vi "Get RPC getCANDatafromrgrpcServer_clientRequester_getIDFormServer __Input.vi"(8 "error in (no error)":errorcluster, 11 "gRPCid in":T1) -> (0 "error out":errorcluster, 2 "Message Data":T2, 3 "gRPCid out":T1)   [LabVIEW 2020, in "server12.lvlib" / "server12.lvclass"]
uses:
  server12.lvclass
  gRPC lvSupport/Server API/typeDefs/grpcId.ctl
  server12.lvclass/server12.ctl
  gRPC lvSupport/gprc-lvsupport.lvlib
  RPC Messages/getCANDatafromrgrpcServer_inputSettings/getCANDatafromrgrpcServer_inputSettings_Data.ctl
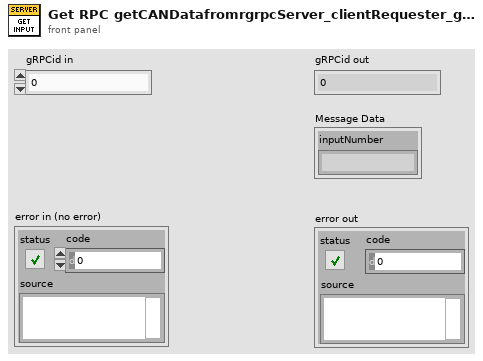
[diagram p1: front panel]
types:
  T1 = typedef "server12.lvlib/gprc-lvsupport.lvlib/grpcId.ctl" = u64
  T2 = typedef "server12.lvlib/server12.lvclass/getCANDatafromrgrpcServer_inputSettings_Data.ctl" = cluster{"inputNumber":string}
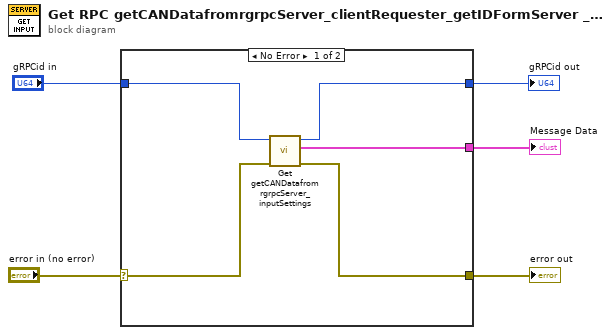
[diagram p0: block diagram]
diagram:
  n1 = case shown="No Error" "error in (no error)" {
    selector: "error in (no error)" -> [w10 w11]
    tunnel: [w9 w11] -> w4
    tunnel: "gRPCid in" -> [w8 w12]
    tunnel: [w7 _] -> w2
    tunnel: [w6 w12] -> w1
    frame No Error {
      n2 = call "Get getCANDatafromrgrpcServer_inputSettings.vi"("error in (no error)"=w10, "gRPCid"=w8) -> ("error out"=w9:errorcluster, "Message Data"=w7:T2, "gRPCid out"=w6:T1)  [unwired: 7 in]
    }
    frame Error {
    }
  }
  "error out" <- w4
  "Message Data" <- w2
  "gRPCid out" <- w1
